vi "CalculateStartupRMSamp.vi"(8 "error in (no error)":errorcluster, 10 "frequency":dbl, 11 "current waveforms":waveform(dbl)[](array[waveform])) -> (0 "error out":errorcluster, 3 "3-phase Max Startup RMS (rms)":sgl)   [LabVIEW 2017, in "McsaAnalysisFunctions.lvlib"]
uses:
  <vilib>/addons/InsightCM/Utilities/Analysis/MCSA/McsaAnalysisFunctions.lvlib
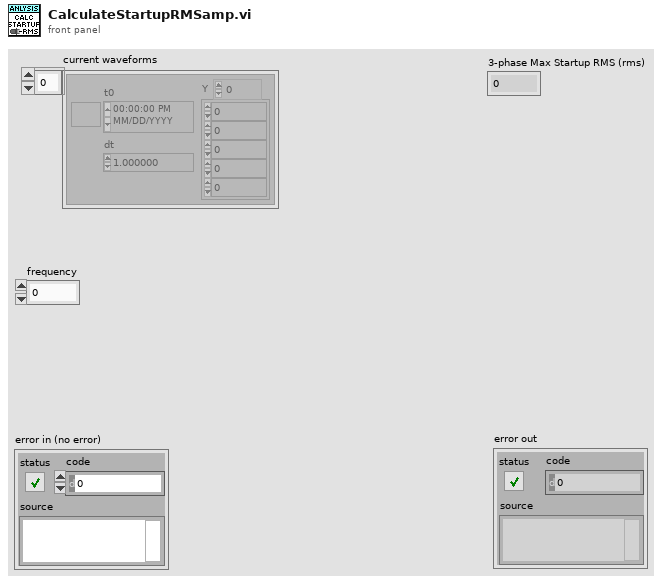
[diagram p1: front panel]
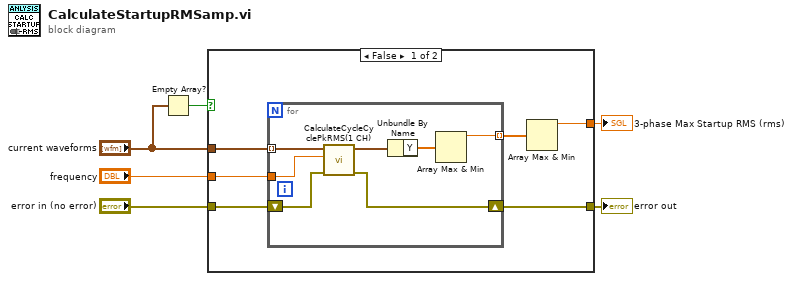
[diagram p0: block diagram]
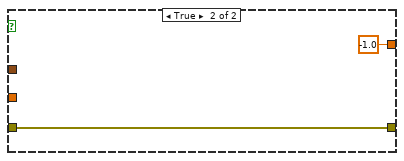
[diagram p2: hidden frame]
diagram:
  n1 = Empty Array?(array="current waveforms") -> (empty?=w2:bool)
  n2 = case shown="False" w2 {
    tunnel: "current waveforms" -> [w12 _]
    tunnel: "error in (no error)" -> [w11 w20]
    tunnel: [w10 w20] -> w5
    tunnel: [w8 sgl -1.0] -> w4
    tunnel: "frequency" -> [w7 _]
    frame False {
      n3 = for {
        tunnel: w12 -> [w19] mode=indexing
        tunnel: w7 -> [w18]
        shift-right: [w16] -> w10
        shift-left: w11 -> [w17]
        tunnel: [w13] -> w9 mode=indexing
        n4 = call <vilib>:"CalculateCycleCyclePkRMS(1 CH).vi"("error in (no error)"=w17, "line frequency"=w18, "waveform"=w19) -> ("error out"=w16:errorcluster, "rms waveform"=w14:waveform(dbl))  [unwired: 6 in, 1 out]
        n5 = Unbundle By Name(w14) -> ("Y"=w15:dbl[])
        n6 = Array Max & Min(array=w15) -> (max value=w13:dbl)  [unwired: 3 out]
      }
      n7 = Array Max & Min(array=w9) -> (max value=w8:dbl)  [unwired: 3 out]
    }
    frame True {
    }
  }
  "error out" <- w5
  "3-phase Max Startup RMS (rms)" <- w4
